vi "tsdiag_can_request_upload.vi"(6 "AMemSize":u32, 8 "error in (no error)":errorcluster, 9 "AMemAddr":u32, 10 "ADiagModuleIndex":i32, 11 "路径输入":path) -> (0 "error out":errorcluster, 2 "return":i32, 3 "路径输出":path)   [LabVIEW 2014]
doc: "35服务，请求上传数据。"
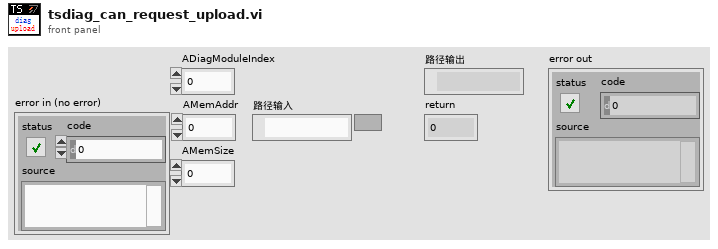
[diagram p1: front panel]
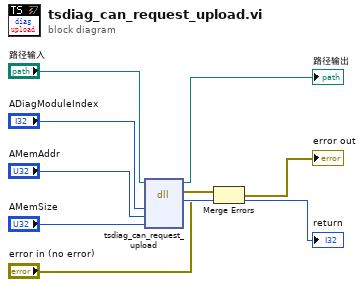
[diagram p0: block diagram]
diagram:
  n1 = dll-call lib="D:/Program Files (x86)/TOSUN/TSMaster/bin/TSMaster.dll" fn="tsdiag_can_request_upload"(path in="路径输入", "ADiagModuleIndex"="ADiagModuleIndex", "AMemAddr"="AMemAddr", "AMemSize"="AMemSize") -> (path out=→"路径输出":path, error out=w9:errorcluster, "ACode"=→"return":i32)  [unwired: 5 in]
  n2 = Merge Errors(w9, "error in (no error)") -> (→"error out":errorcluster)
